vi "Register for Draw Tree.vi"(8 "error in (no error)":errorcluster, 11 "Process Explorer View in":refnum<class "Process Explorer View.lvclass">) -> (0 "error out":errorcluster, 3 "Process Explorer View out":refnum<class "Process Explorer View.lvclass">)   [LabVIEW 2019, in "Process Explorer View.lvclass"]
uses:
  <vilib>/gpm_packages/@cs/Car-wash/Source/Process Explorer View/Process Explorer View.lvclass
  C:/Program Files/National Instruments/LabVIEW 2019/vi.lib/gpm_packages/@cs/mva-core/Source/IObserver/IObserver/IObserver.lvclass
  <vilib>/gpm_packages/@cs/file-explorer-extension/Source/File Explorer/File Explorer Messages/Draw Tree Control Msg/Draw Tree Control Msg.lvclass
  C:/Program Files/National Instruments/LabVIEW 2019/vi.lib/gpm_packages/@cs/transport/Source/Concrete/ActorMessageTransport/Notification Msg/Notification Msg.lvclass
  <vilib>/gpm_packages/@cs/mva-core/Source/SubscriptionPolicy/BasicSubscription/BasicSubscription.lvclass/BasicSubscription.ctl
  <vilib>/ActorFramework/Actor/Actor.lvclass/Actor.ctl
  <vilib>/ActorFramework/Message Enqueuer/Message Enqueuer.lvclass/Message Enqueuer.ctl
  <vilib>/gpm_packages/@cs/transport/Source/Concrete/ActorMessageTransport/ActorMessageTransport.lvclass/ActorMessageTransport.ctl
  <vilib>/gpm_packages/@cs/mva-core/Source/IMediator/SubscriptionRequest/SubscriptionRequest.lvclass/SubscriptionRequest.ctl
  <vilib>/gpm_packages/@cs/mva-core/Source/IObserver/IObserver Messages/Subscribe Msg/Subscribe Msg.lvclass/Subscribe Msg.ctl
  <vilib>/gpm_packages/@cs/mva-core/Source/IMediator/SubscriptionRequest/Pack Subscription Request.vi
  <vilib>/gpm_packages/@cs/mva-core/Source/IObserver/IObserver Messages/Subscribe Msg/Send Subscribe.vi
  <vilib>/ActorFramework/Actor/Read Self Enqueuer.vi
  <vilib>/gpm_packages/@cs/transport/Source/Concrete/ActorMessageTransport/Construct Actor Message Transport.vi
  <vilib>/ActorFramework/Message Enqueuer/Enqueue.vi
  <vilib>/ActorFramework/Message Enqueuer/Init from Existing Queue.vi
  <vilib>/ActorFramework/Message Enqueuer/Equals Not A Refnum.vi
  <vilib>/gpm_packages/@cs/mva-core/Source/SubscriptionPolicy/BasicSubscription/BasicSubscription.lvclass
  C:/Program Files/National Instruments/LabVIEW 2019/vi.lib/gpm_packages/@cs/mva-core/Source/IMediator/ISubscriptionPolicy/ISubscriptionPolicy.lvclass
  <vilib>/gpm_packages/@cs/mva-core/Source/IObserver/IObserver/IObserver.lvclass
  C:/Program Files/National Instruments/LabVIEW 2019/vi.lib/ActorFramework/Actor/Actor.lvclass
  <vilib>/gpm_packages/@cs/transport/Source/Concrete/ActorMessageTransport/ActorMessageTransport.lvclass
  C:/Program Files/National Instruments/LabVIEW 2019/vi.lib/gpm_packages/@cs/transport/Source/ITransport/ITransport.lvclass
  <vilib>/gpm_packages/@cs/mva-core/Source/IObserver/IObserver Messages/Subscribe Msg/Subscribe Msg.lvclass
  C:/Program Files/National Instruments/LabVIEW 2019/vi.lib/ActorFramework/Message/Message.lvclass
  <vilib>/Utility/error.llb/Error Cluster From Error Code.vi
  <vilib>/gpm_packages/@cs/mva-core/Source/IMediator/ISubscriptionPolicy/Open Subscription Policy.vi
  <vilib>/ActorFramework/Message Priority Queue/Priority Enqueue.vi
  <vilib>/ActorFramework/Message Enqueuer/Message Enqueuer.lvclass
  <vilib>/gpm_packages/@cs/mva-core/Source/IMediator/SubscriptionRequest/SubscriptionRequest.lvclass
  <vilib>/gpm_packages/@cs/transport/Source/Concrete/ActorMessageTransport/Notification Msg/Notification Msg.lvclass
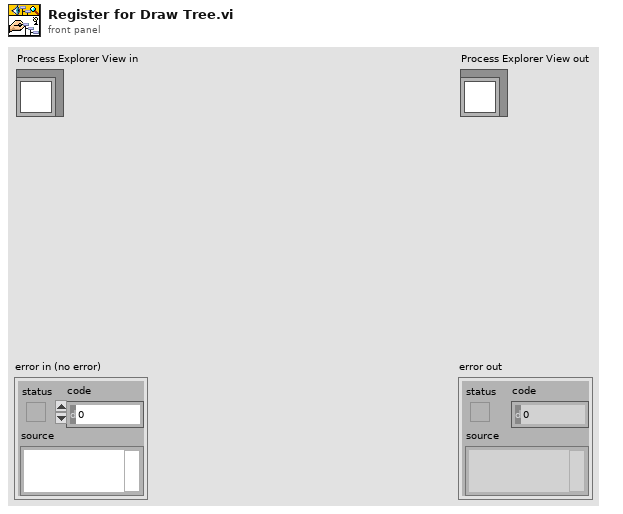
[diagram p1: front panel]
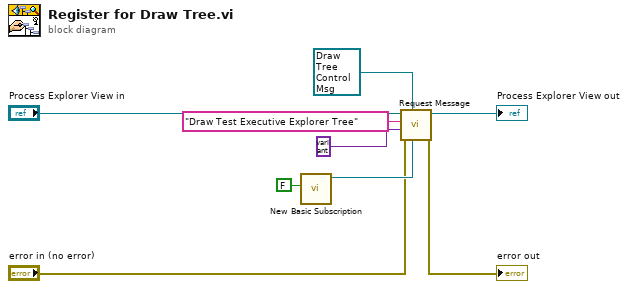
[diagram p0: block diagram]
diagram:
  n1 = call <vilib>:"New Basic Subscription.vi"("Ignore Past Updates? (F)"=FALSE) -> ("BasicSubscription Out"=w6:refnum<class "BasicSubscription.lvclass">)  [unwired: 10 in]
  n2 = call <vilib>:"Request Message.vi"("Configured SubscriptionPolicy"=w6, "Desired Notification Msg"=refnum<class "Draw Tree Control Msg.lvclass"> refnum ("File Explorer.lvlib:Draw Tree Control Msg.lvclass"), "error in (no error)"="error in (no error)", "Data Type"=variant, "Datum Name"="Draw Test Executive Explorer Tree", "IObserver in"="Process Explorer View in") -> ("error out"=→"error out":errorcluster, "IObserver out"=→"Process Explorer View out":refnum<class "Process Explorer View.lvclass">)  [unwired: 3 in, 1 out]
